vi "Open Path File.vi"(11 "File Name":string) -> (3 "Trajectory Data":T1(array[cluster]))   [LabVIEW 2019]
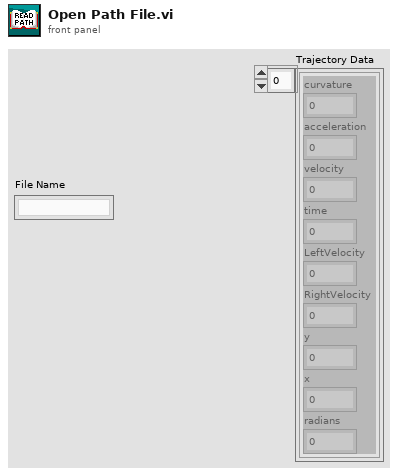
[diagram p1: front panel]
types:
  T1 = cluster{"curvature":dbl, "acceleration":dbl, "velocity":dbl, "time":dbl, "LeftVelocity":dbl, "RightVelocity":dbl, "y":dbl, "x":dbl, "radians":dbl}[]
  T2 = cluster{"curvature":dbl, "acceleration":dbl, "velocity":dbl, "time":dbl, "LeftVelocity":dbl, "RightVelocity":dbl, "y":dbl, "x":dbl, "radians":dbl}
  T3 = enum16{"open", "replace", "create", "open or create", "replace or create", "replace or create with confirmation"}
  T4 = cluster{"pose":cluster{"rotation":cluster{"radians":dbl}}}[]
  T5 = cluster{"pose":cluster{"translation":cluster{"y":dbl, "x":dbl}}}[]
  T6 = cluster{"curvature":dbl, "acceleration":dbl, "velocity":dbl, "time":dbl}[]
  T7 = cluster{"curvature":dbl, "acceleration":dbl, "velocity":dbl, "time":dbl}
  T8 = cluster{"pose":cluster{"translation":cluster{"y":dbl, "x":dbl}}}
  T9 = cluster{"pose":cluster{"rotation":cluster{"radians":dbl}}}
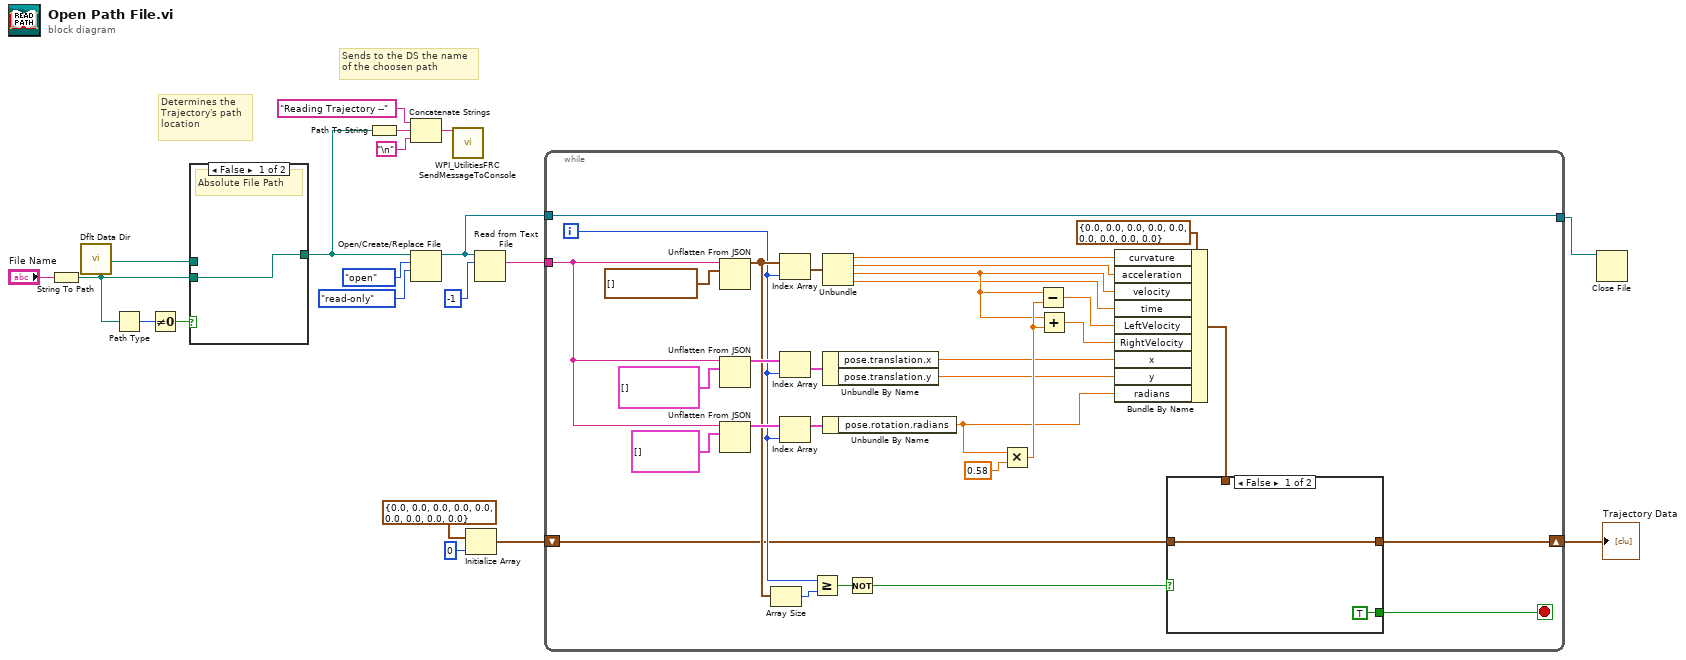
[diagram p0: block diagram]
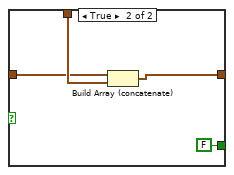
[diagram p2: hidden frame]
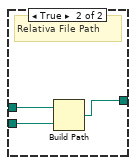
[diagram p3: hidden frame]
diagram:
  # "Sends to the DS the name\nof the choosen path"
  # "Determines the \nTrajectory's path \nlocation"
  n1 = String To Path(string="File Name") -> (path=w16:path)
  n2 = call <vilib>:"Dflt Data Dir.vi"() -> ("App:Default Data Directory"=w20:path)
  n3 = Path Type(1:w16) -> (0:w17:i16)
  n4 = Not Equal To 0?(x=w17) -> (x != 0?=w18:bool)
  n5 = case shown="False" w18 {
    tunnel: [w21 w24] -> w12
    tunnel: w20 -> [_ w23]
    tunnel: w16 -> [w21 w22]
    frame False {
      # "Absolute File Path"
    }
    frame True {
      # "Relativa File Path"
      n6 = Build Path(base path=w23, name or relative path=w22) -> (appended path=w24:path)
    }
  }
  n7 = Path To String(path=w12) -> (string=w11:string)
  n8 = Concatenate Strings("Reading Trajectory --" ("string"), w11, "\n") -> (w9:string)
  n9 = Open/Create/Replace File(file path (use dialog)=w12, operation (0:open)=T3."open", access (0:read/write)=enum16{"read/write", "read-only", "write-only"}."read-only") -> (refnum out=w2:refnum<file>)  [unwired: 3 in, 2 out]
  n10 = call <vilib>:"WPI_UtilitiesFRC SendMessageToConsole.vi"("Message"=w9) -> ()  [unwired: 14 in, 1 out]
  n11 = Initialize Array(T2 {"curvature"=0.0, "acceleration"=0.0, "velocity"=0.0, "time"=0.0, "LeftVelocity"=0.0, "RightVelocity"=0.0, "y"=0.0, "x"=0.0, "radians"=0.0}, 0 ("dimension size")) -> (w4:T1)
  n12 = Read from Text File(file (use dialog)=w2, count=-1) -> (text=w7:string)  [unwired: 2 in, 3 out]
  n13 = while {
    tunnel: w7 -> [w47]
    shift-right: [w26] -> w3
    shift-left: w4 -> [w27]
    tunnel: w2 -> [w25]
    tunnel: [w25] -> w1
    i -> [w42]
    stop <- w28 stop-if-true
    n14 = Unflatten From JSON(JSON string=w47, type and defaults=T6 []) -> (value=w44:T6)  [unwired: 5 in, 1 out]
    n15 = Unflatten From JSON(JSON string=w47, type and defaults=T5 []) -> (value=w53:T5)  [unwired: 5 in, 1 out]
    n16 = Unflatten From JSON(JSON string=w47, type and defaults=T4 []) -> (value=w54:T4)  [unwired: 5 in, 1 out]
    n17 = Array Size(array=w44) -> (size(s)=w43:i32)
    n18 = Index Array(array=w44, index=w42) -> (element=w55:T7)
    n19 = Index Array(array=w53, index=w42) -> (element=w52:T8)
    n20 = Index Array(array=w54, index=w42) -> (element=w51:T9)
    n21 = Greater Or Equal?(x=w42, y=w43) -> (x >= y?=w30:bool)
    n22 = Unbundle(w55) -> ("curvature"=w35:dbl, "acceleration"=w34:dbl, "velocity"=w33:dbl, "time"=w32:dbl)
    n23 = Unbundle By Name(w52) -> ("pose.translation.x"=w40:dbl, "pose.translation.y"=w39:dbl)
    n24 = Unbundle By Name(w51) -> ("pose.rotation.radians"=w38:dbl)
    n25 = Not(x=w30) -> (.not. x?=w29:bool)
    n26 = Multiply(x=w38, y=0.58) -> (x*y=w45:dbl)
    n27 = Subtract(x=w33, y=w45) -> (x-y=w36:dbl)
    n28 = Add ("Right Wheel Velocity")(x=w33, y=w45) -> (x+y=w37:dbl)
    n29 = Bundle By Name(cluster=T2 {"curvature"=0.0, "acceleration"=0.0, "velocity"=0.0, "time"=0.0, "LeftVelocity"=0.0, "RightVelocity"=0.0, "y"=0.0, "x"=0.0, "radians"=0.0}, "curvature"=w35, "acceleration"=w34, "velocity"=w33, "time"=w32, "LeftVelocity"=w36, "RightVelocity"=w37, "x"=w40, "y"=w39, "radians"=w38) -> (w31:T2)
    n30 = case shown="False" w29 {
      tunnel: w31 -> [_ w61]
      tunnel: [TRUE FALSE] -> w28
      tunnel: w27 -> [w56 w59]
      tunnel: [w56 w58] -> w26
      frame False {
      }
      frame True {
        n31 = Build Array (concatenate)(w59, w61) -> (w58:T1)
      }
    }
  }
  "Trajectory Data" <- w3
  n32 = Close File(refnum=w1) -> ()  [unwired: 1 in, 2 out]
